vi "LendoAgilent.vi"() -> ()   [LabVIEW 2019]
uses:
  <instrlib>/Agilent 34970/Agilent 34970.lvlib
panel:
  out "Waveform Chart":dbl(graph)
  in  "stop":bool
  out "Output Array":dbl[](array[numeric]) format="%.2f"
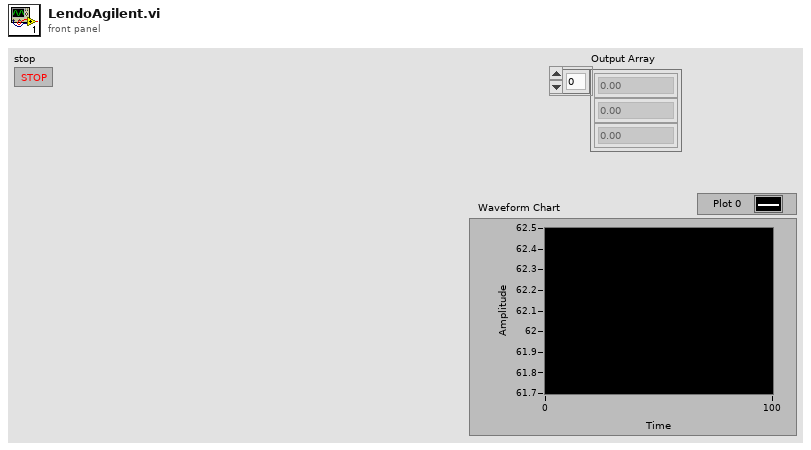
[diagram p1: front panel]
types:
  T1 = enum16{"Thermocouple", "Thermistor", "RTD", "4-Wire RTD", "Default (Last)"}
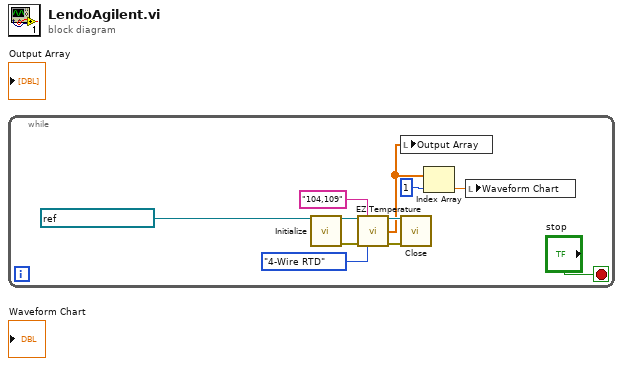
[diagram p0: block diagram]
diagram:
  n1 = while {
    stop <- "stop" stop-if-true
    n2 = call <instrlib>:"Initialize.vi"("VISA Resource Name"=refnum<visa-resource-name> "A-34972A-06789") -> ("VISA Resource Name Out"=w7:refnum<visa-resource-name>, "error out"=w8:errorcluster)  [unwired: 13 in]
    n3 = call <instrlib>:"EZ Temperature.vi"("VISA Resource Name"=w7, "Scan List (empty)"="104,109", "error in (no error)"=w8, "Transducer Type (4:Def-Last)"=T1."4-Wire RTD") -> ("VISA Resource Name Out"=w10:refnum<visa-resource-name>, "Output Array"=w3:dbl[], "error out"=w9:errorcluster)  [unwired: 9 in]
    n4 = local write "Output Array"(w3) -> ()
    n5 = call <instrlib>:"Close.vi"("VISA Resource Name"=w10, "error in (no error)"=w9) -> ()  [unwired: 13 in, 1 out]
    n6 = Index Array(array=w3, index=1) -> (element=w1:dbl)
    n7 = local write "Waveform Chart"(w1) -> ()
  }
